vi "Change DAQ Parameter.vi"(8 "error in":errorcluster, 11 "tCRD in":refnum<class "Open Path CRD.lvclass">) -> (0 "error out":errorcluster, 3 "tCRD out":refnum<class "Open Path CRD.lvclass">)   [LabVIEW 2015, in "Open Path CRD.lvclass"]
doc: "Change the sample time (period over which we acquire data) and the rate at which we acquire data if requested."
uses:
  Open Path CRD.lvclass
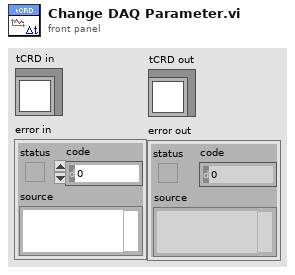
[diagram p1: front panel]
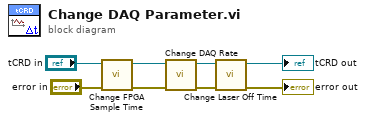
[diagram p0: block diagram]
diagram:
  n1 = call "Change FPGA Sample Time.vi"("error in"="error in", "tCRD in"="tCRD in") -> ("error out"=w6:errorcluster, "tCRD out"=w8:refnum<class "Open Path CRD.lvclass">)  [unwired: 8 in]
  n2 = call "Change DAQ Rate.vi"("error in (no error)"=w6, "tCRD in"=w8) -> ("error out"=w2:errorcluster, "tCRD out"=w5:refnum<class "Open Path CRD.lvclass">)  [unwired: 8 in]
  n3 = call "Change Laser Off Time.vi"("error in"=w2, "tCRD in"=w5) -> ("error out"=→"error out":errorcluster, "tCRD out"=→"tCRD out":refnum<class "Open Path CRD.lvclass">)  [unwired: 8 in]
